vi "insert or remove.vi"(6 "replace entry if exists":bool, 7 "action":T2, 8 "error in (no error)":errorcluster, 10 "entry":T1, 11 "id":string) -> (0 "error out":errorcluster)   [LabVIEW 2024, in "status manager.lvlib"]
uses:
  status manager.lvlib
  insert or remove.ctl
  entry type.ctl
  fgv actions.ctl
  <vilib>/Utility/error.llb/Error Cluster From Error Code.vi
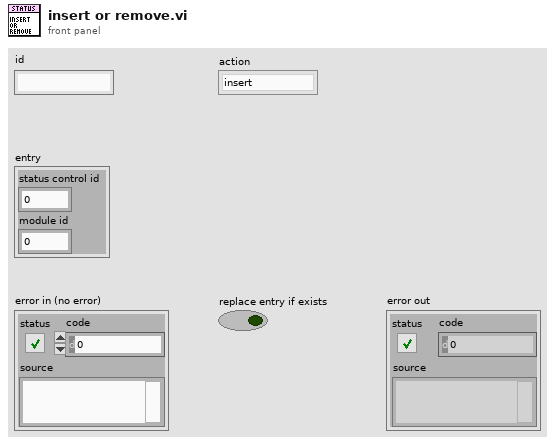
[diagram p1: front panel]
types:
  T1 = typedef "status manager.lvlib/entry type.ctl" = cluster{"status control id":i32, "module id":i32}
  T2 = typedef "status manager.lvlib/insert or remove.ctl" = enum16{"insert", "remove"}
  T3 = typedef "status manager.lvlib/fgv actions.ctl" = enum16{"create", "get", "destroy"}
  T4 = typedef "status manager.lvlib/collection type.ctl" = map{string, T1}
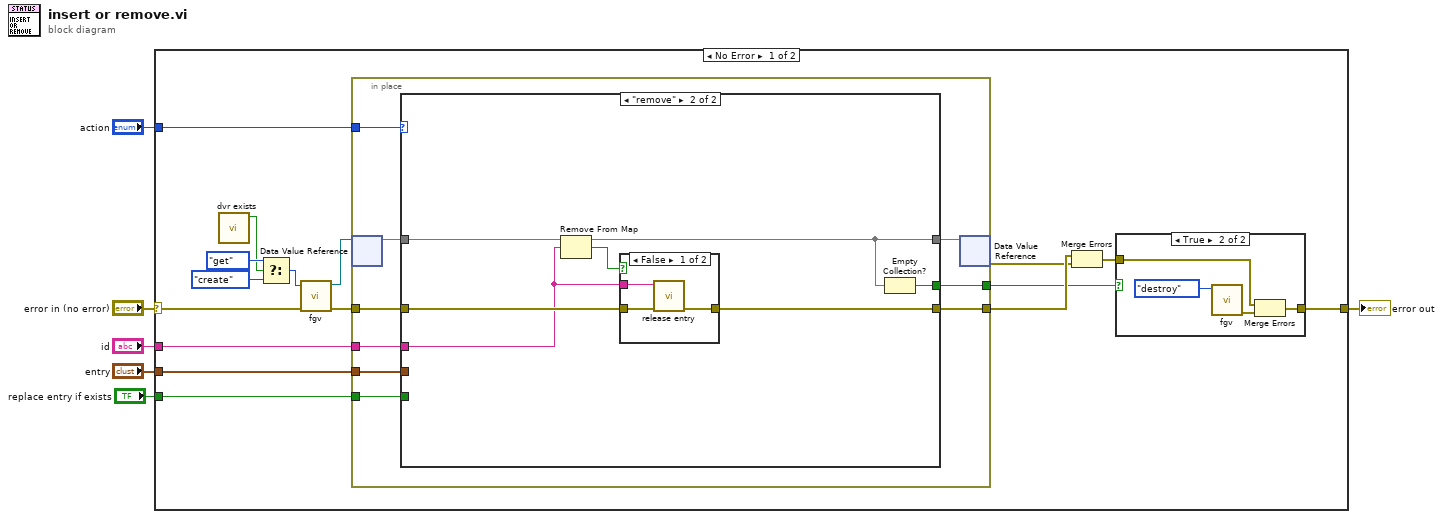
[diagram p0: block diagram]
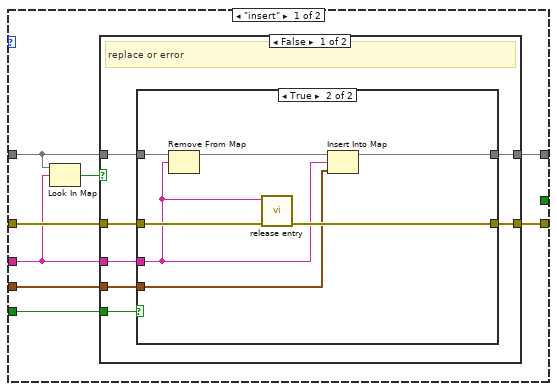
[diagram p2: hidden frame]
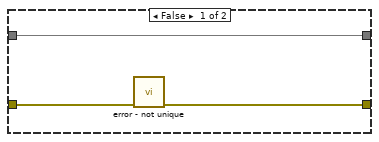
[diagram p3: hidden frame]
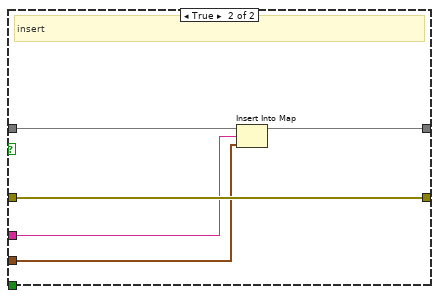
[diagram p4: hidden frame]
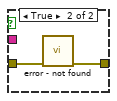
[diagram p5: hidden frame]
diagram:
  n1 = case shown="No Error" "error in (no error)" {
    selector: "error in (no error)" -> [w10 w79]
    tunnel: "replace entry if exists" -> [w22 _]
    tunnel: [w18 w79] -> w4
    tunnel: "entry" -> [w12 _]
    tunnel: "action" -> [w17 _]
    tunnel: "id" -> [w11 _]
    frame No Error {
      n2 = call "dvr exists.vi"() -> ("exists"=w7:bool)  [unwired: 10 in, 1 out]
      n3 = Select(t=fgv_actions."get", s=w7, f=fgv_actions."create") -> (s? t:f=w14:T3)
      n4 = call "fgv.vi"("error in (no error)"=w10, "action"=w14) -> ("error out"=w9:errorcluster, "dvr"=w16:refnum<data-value>)  [unwired: 8 in]
      n5 = in-place {
        in-place-border: [w29] -> w8
        in-place-border: w12 -> [w28]
        in-place-border: w22 -> [w27]
        in-place-border: w9 -> [w26]
        in-place-border: [w25] -> w21
        in-place-border: w11 -> [w24]
        in-place-border: w17 -> [w23]
        n6 = in-place-dvr #1(w16) -> (w31:T4)  [unwired: 1 out]
        n7 = case shown="\"remove\"" w23 {
          tunnel: w31 -> [w33 w64]
          tunnel: [w32 w63] -> w30
          tunnel: [_ w68] -> w29
          tunnel: w28 -> [w39 _]
          tunnel: w27 -> [w38 _]
          tunnel: w26 -> [w37 w67]
          tunnel: [w36 w66] -> w25
          tunnel: w24 -> [w35 w62]
          frame "insert" {
            n8 = Look In Map(map=w33, key=w35) -> (key not found?=w34:bool)  [unwired: 1 in, 1 out]
            n9 = case shown="False" w34 {
              tunnel: [w43 w60] -> w32
              tunnel: w33 -> [w45 w59]
              tunnel: w39 -> [w44 w58]
              tunnel: w38 -> [w46 _]
              tunnel: w37 -> [w42 w61]
              tunnel: [w41 w61] -> w36
              tunnel: w35 -> [w40 w57]
              frame False {
                # "replace or error"
                n10 = case shown="True" w46 {
                  tunnel: w45 -> [w49 w55]
                  tunnel: w44 -> [_ w53]
                  tunnel: [w49 w52] -> w43
                  tunnel: w42 -> [w48 w51]
                  tunnel: [w47 w56] -> w41
                  tunnel: w40 -> [_ w50]
                  frame False {
                    n11 = call "error - not unique.vi"("error in (no error)"=w48) -> ("error out"=w47:errorcluster)  [unwired: 10 in]
                  }
                  frame True {
                    n12 = Remove From Map(10:w50, 11:w55) -> (3:w54:T4)  [unwired: 2 out]
                    n13 = call "release entry.vi"("error in (no error)"=w51, "id"=w50) -> ("error out"=w56:errorcluster)  [unwired: 9 in]
                    n14 = Insert Into Map(map in=w54, key=w50, value=w53) -> (map out=w52:T4)  [unwired: 2 out]
                  }
                }
              }
              frame True {
                # "insert"
                n15 = Insert Into Map(map in=w59, key=w57, value=w58) -> (map out=w60:T4)  [unwired: 2 out]
              }
            }
          }
          frame "remove" {
            n16 = Remove From Map(10:w62, 11:w64) -> (2:w65:bool, 3:w63:T4)  [unwired: 1 out]
            n17 = case shown="False" w65 {
              tunnel: w62 -> [w71 _]
              tunnel: w67 -> [w70 w73]
              tunnel: [w69 w72] -> w66
              frame False {
                n18 = call "release entry.vi"("error in (no error)"=w70, "id"=w71) -> ("error out"=w69:errorcluster)  [unwired: 9 in]
              }
              frame True {
                n19 = call "error - not found.vi"("error in (no error)"=w73) -> ("error out"=w72:errorcluster)  [unwired: 10 in]
              }
            }
            n20 = Empty Collection?(1:w63) -> (0:w68:bool)
          }
        }
        n21 = in-place-dvr #1(w30) -> (w20:errorcluster)  [unwired: 1 out]
      }
      n22 = Merge Errors(w21, w20) -> (w19:errorcluster)
      n23 = case shown="True" w8 {
        tunnel: w19 -> [w74 w77]
        tunnel: [w74 w78] -> w18
        frame False {
        }
        frame True {
          n24 = call "fgv.vi"("action"=fgv_actions."destroy") -> ("error out"=w75:errorcluster)  [unwired: 9 in, 1 out]
          n25 = Merge Errors(w77, w75) -> (w78:errorcluster)
        }
      }
    }
    frame Error {
    }
  }
  "error out" <- w4
